vi "DSF.Engine.Interface.Set Response FIFO.vi"(10 "Response FIFO":T1, 11 "Interface in":refnum<class "DSF.Engine.Interface.lvclass">) -> (3 "Interface out":refnum<class "DSF.Engine.Interface.lvclass">)   [LabVIEW 2017, in "Data Sharing Framework Engine.lvlib" / "DSF.Engine.Interface.lvclass"]
uses:
  DSF.Engine.Interface.lvclass
  DSF.Engine.Interface.RT FIFO.Ref.16B.ctl
  DSF.Engine.Interface.RT FIFO.Data.16B.ctl
  DSF.Engine.Interface.RT FIFO.Payload.16B.ctl
  DSF.Engine.Interface.lvclass/DSF.Engine.Interface.ctl
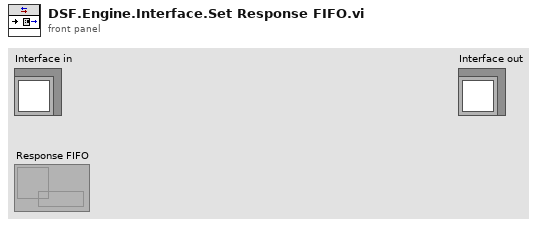
[diagram p1: front panel]
types:
  T1 = typedef "Data Sharing Framework Engine.lvlib/DSF.Engine.Interface.lvclass/DSF.Engine.Interface.RT FIFO.Ref.16B.ctl" = refnum<k33>
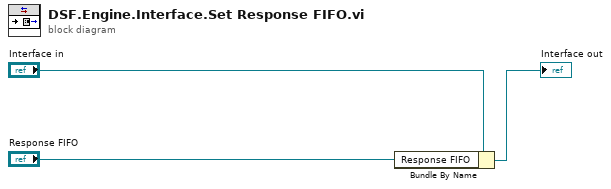
[diagram p0: block diagram]
diagram:
  n1 = Bundle By Name(cluster="Interface in", "Response FIFO"="Response FIFO") -> (→"Interface out":refnum<class "DSF.Engine.Interface.lvclass">)
